vi "AMI1700_meas_he_lev.vi"(8 "error in":errorcluster, 11 "VISA in":refnum<visa-resource-name>) -> (0 "error out":errorcluster, 1 "level":dbl, 2 "status":bool, 3 "VISA out":refnum<visa-resource-name>)   [LabVIEW 2019]
uses:
  <vilib>/numeric/Random Number (Range) DBL.vi
panel:
  out "string 2":string
  out "string 1":string
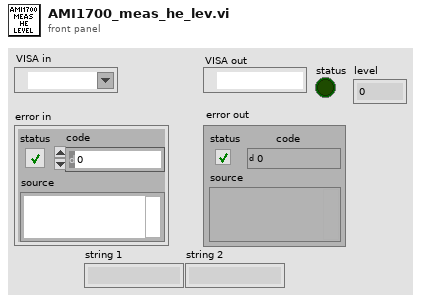
[diagram p1: front panel]
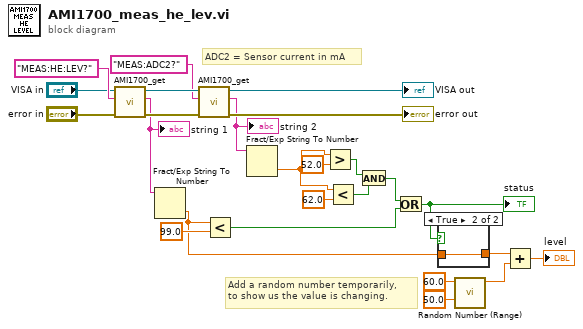
[diagram p0: block diagram]
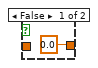
[diagram p2: hidden frame]
diagram:
  # "Add a random number temporarily,\nto show us the value is changing."
  # "ADC2 = Sensor current in mA"
  n1 = call "AMI1700_get.vi"("error in"="error in", "string in"="MEAS:HE:LEV?" ("string"), "VISA in"="VISA in") -> ("error out"=w20:errorcluster, "string out"=w10:string, "VISA out"=w22:refnum<visa-resource-name>)  [unwired: 6 in]
  "string 1" <- w10
  n2 = Fract/Exp String To Number(string=w10) -> (number=w6:dbl)  [unwired: 3 in, 1 out]
  n3 = call "AMI1700_get.vi"("error in"=w20, "string in"="MEAS:ADC2?" ("string"), "VISA in"=w22) -> ("error out"=→"error out":errorcluster, "string out"=w17:string, "VISA out"=→"VISA out":refnum<visa-resource-name>)  [unwired: 6 in]
  "string 2" <- w17
  n4 = Less?(x=w6, y=99.0) -> (x < y?=w8:bool)
  n5 = Fract/Exp String To Number(string=w17) -> (number=w12:dbl)  [unwired: 3 in, 1 out]
  n6 = Greater?(x=w12, y=52.0) -> (0:w14:bool)
  n7 = Less?(x=w12, y=62.0) -> (x < y?=w13:bool)
  n8 = And(x=w14, y=w13) -> (x .and. y?=w9:bool)
  n9 = Or(x=w9, y=w8) -> (x .or. y?=w7:bool)
  "status" <- w7
  n10 = case shown="True" w7 {
    tunnel: [0.0 w27] -> w5
    tunnel: w6 -> [_ w27]
    frame False {
    }
    frame True {
    }
  }
  n11 = call-poly <vilib>:"Random Number (Range).vi"("lower bound (0)"=50.0, "upper bound (100)"=60.0) -> ("number"=w1:dbl)  [unwired: 9 in]
  n12 = Add(x=w5, y=w1) -> (x+y=→"level":dbl)
